vi "SimpleExample1_DS_server.vi"() -> ()   [LabVIEW 2011, in "Messenging.lvlib"]
uses:
  Messenging.lvlib
  Interprocess Messenger/TextVarientMessage/MSG.lvclass
  Interprocess Messenger/TextVarientMessage/Reply (varient).vi
  Interprocess Messenger/DataSocketMessenger/DataSocketMessenger.lvclass
panel:
  out "net address":u32
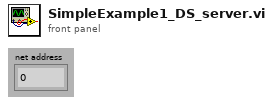
[diagram p1: front panel]
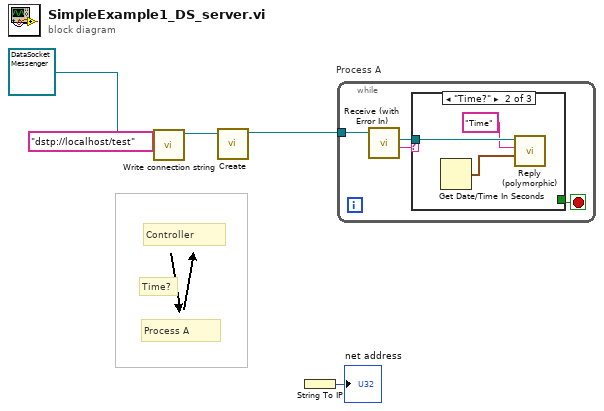
[diagram p0: block diagram]
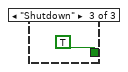
[diagram p3: hidden frame]
diagram:
  # "Time?"
  # "Process A"
  # "Controller"
  n1 = call-dynamic "Write connection string.vi"("connection string"="dstp://localhost/test", "DataSocketMessenger.lvclass in"=refnum<class "DataSocketMessenger.lvclass"> refnum ("Messenging.lvlib:DataSocketMessenger.lvclass")) -> ("DataSocketMessenger.lvclass out"=w2:refnum<class "DataSocketMessenger.lvclass">)  [unwired: 1 in, 8 out]
  n2 = call-dynamic "Create.vi"("DataSocketMessenger in"=w2) -> ("DataSocketMessenger out"=w5:refnum<class "DataSocketMessenger.lvclass">)  [unwired: 1 in, 9 out]
  n3 = String To IP() -> (0:→"net address":u32)  [unwired: 1 out]
  n4 = while "Process A" {
    tunnel: w5 -> [w9]
    stop <- w6 stop-if-true
    n5 = call-dynamic "Receive (with Error In).vi"("MGR in"=w9) -> ("Label"=w8:string, "Message"=w7:refnum<class "MSG.lvclass">)  [unwired: 2 in, 7 out]
    n6 = case shown="\"Time?\"" w8 {
      tunnel: w7 -> [_ w12 _]
      tunnel: [_ _ TRUE] -> w6
      frame "False", Default {
      }
      frame "Time?" {
        n7 = Get Date/Time In Seconds() -> (seconds since 1Jan1904=w11:timestamp)
        n8 = call-poly "Reply (polymorphic).vi"("Varient"=w11, "Reply"="Time", "Message to Reply to"=w12) -> ()  [unwired: 1 in, 8 out]
      }
      frame "Shutdown" {
      }
    }
  }
